vi "Test_Drive_Motor.vi"() -> ()   [LabVIEW 2019]
uses:
  <vilib>/myRIO/Instrument Drivers/Onboard IO/DIO/typedefs/DIO Reference.ctl
  <vilib>/myRIO/Common/Instrument Driver Framework/Utilities/typedefs/myRIO Generic Hardware Reference.ctl
  <vilib>/myRIO/Common/Instrument Driver Framework/Utilities/typedefs/Hardware Version Enum.ctl
  <vilib>/myRIO/Common/Instrument Driver Framework/Utilities/typedefs/myRIO v1.0 Reference.ctl
  <vilib>/myRIO/Common/Instrument Driver Framework/Utilities/typedefs/Generic FPGA Reference.ctl
  <vilib>/myRIO/Common/Instrument Driver Framework/myRIO v1.0/DIO/typedefs/DIO Channels List.ctl
  <vilib>/myRIO/Common/Instrument Driver Framework/myRIO v1.0/DIO/typedefs/DIO Channels Enum.ctl
  <vilib>/userDefined/High Color/nirio_resource_hc.ctl
  L298N_Driver/L298N_Ref_Type.ctl
  L298N_Driver/L298N_Action_Enum.ctl
  <vilib>/myRIO/Common/Instrument Driver Framework/myRIO v1.0/DIO/vis/myRIO v1.1 Open DIO.vi
  <vilib>/myRIO/Common/Instrument Driver Framework/Utilities/vis/Validate Channels.vi
  <vilib>/myRIO/Common/Instrument Driver Framework/myRIO v1.0/DIO/vis/myRIO v1.0 Reserve DIO.vi
  <vilib>/myRIO/Common/Instrument Driver Framework/myRIO v1.0/DIO/vis/myRIO v1.0 Close DIO.vi
  <vilib>/myRIO/Common/Instrument Driver Framework/myRIO v1.0/Resource Manager/vis/myRIO v1.0 Reserve Channel List.vi
  <vilib>/myRIO/Common/Instrument Driver Framework/myRIO v1.0/DIO/vis/myRIO v1.0 Build MUX Configuration DIO.vi
  <vilib>/myRIO/Common/Instrument Driver Framework/myRIO v1.0/DIO/vis/myRIO v1.0 Unreserve DIO.vi
  <vilib>/myRIO/Common/Instrument Driver Framework/myRIO v1.0/Resource Manager/vis/myRIO v1.0 Reserve Channel.vi
  <vilib>/myRIO/Common/Instrument Driver Framework/myRIO v1.0/Resource Manager/vis/myRIO v1.0 Unreserve Channel.vi
  <vilib>/myRIO/Common/Instrument Driver Framework/myRIO v1.0/Resource Manager/vis/myRIO v1.0 Create Configuration List.vi
  <vilib>/myRIO/Common/Instrument Driver Framework/myRIO v1.0/Resource Manager/vis/myRIO v1.0 Unreserve Channel List.vi
  <vilib>/myRIO/Common/Instrument Driver Framework/myRIO v1.0/Resource Manager/vis/myRIO v1.0 Build Mutex Name.vi
  <vilib>/Utility/VariantDataType/GetNumericInfo.vi
  <vilib>/Utility/error.llb/Error Cluster From Error Code.vi
  <vilib>/myRIO/Common/Instrument Driver Framework/myRIO v1.0/myRIO v1.1 Open.vi
  <vilib>/myRIO/Common/Instrument Driver Framework/Utilities/vis/IO Manager.vi
  <vilib>/myRIO/Common/Instrument Driver Framework/Utilities/vis/Configuration Manager.vi
  <vilib>/myRIO/Common/Instrument Driver Framework/myRIO v1.0/Resource Manager/vis/myRIO v1.0 Configure IO.vi
  <vilib>/myRIO/Common/Instrument Driver Framework/myRIO v1.0/myRIO v1.0 Close.vi
  <vilib>/myRIO/Common/Instrument Driver Framework/myRIO v1.0/DIO/vis/myRIO v1.0 Shutdown DIO.vi
  <vilib>/myRIO/Instrument Drivers/Onboard IO/DIO/vis/myRIO DIO Open.xnode
  <vilib>/myRIO/Instrument Drivers/Onboard IO/DIO/DIO.lvlib
panel:
  out "error out":errorcluster caption="sortie d'erreur"
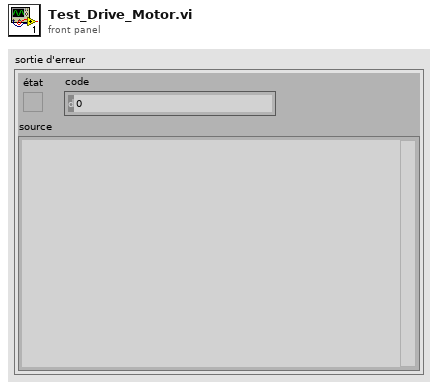
[diagram p1: front panel]
types:
  T1 = typedef "DIO.lvlib/DIO Reference.ctl" = cluster{"myRIO Reference":T2, "DIO Channels List":T6}
  T2 = typedef "myRIO Generic Hardware Reference.ctl" = cluster{"myRIO Model":T3, "myRIO Hardware Reference":T4}
  T3 = typedef "Hardware Version Enum.ctl" = enum16{"Unknown", "myRIO-1900", "myRIO-1950", "roboRIO", "NI ELVIS RIO CM", "ELVIS III"}
  T4 = typedef "myRIO v1.0 Reference.ctl" = cluster{"Generic FPGA Reference":T5, "Allow multiple opens":bool}
  T5 = typedef "Generic FPGA Reference.ctl" = refnum<k20>
  T6 = typedef "DIO Channels List.ctl" = T7[]
  T7 = typedef "DIO Channels Enum.ctl" = enum16{"Not Connected", "C/DIO0", "C/DIO1", "C/DIO2", "C/DIO3", "C/DIO4", "C/DIO5", "C/DIO6", "C/DIO7", "A/DIO0", "A/DIO1", "A/DIO2", "A/DIO3", "A/DIO4", "A/DIO5", "A/DIO6", "A/DIO7", "A/DIO8", "A/DIO9", "A/DIO10", "A/DIO11", "A/DIO12", "A/DIO13", "A/DIO14", "A/DIO15", "A/DIO16", "A/DIO17", "A/DIO18", "A/DIO19", "B/DIO0", "B/DIO1", "B/DIO2", "B/DIO3", "B/DIO4", "B/DIO5", "B/DIO6", "B/DIO7", "B/DIO8", "B/DIO9", "B/DIO10", "B/DIO11", "B/DIO12", "B/DIO13", "B/DIO14", "B/DIO15", "B/DIO16", "B/DIO17", "B/DIO18", "B/DIO19", "LED0", "LED1", "LED2", "LED3", "Button0", "DIO/DIO0", "DIO/DIO1", "DIO/DIO2", "DIO/DIO3", "DIO/DIO4", "DIO/DIO5", "DIO/DIO6", "DIO/DIO7", "DIO/DIO8", "DIO/DIO9", "SPI/CS0", "SPI/CS1", "SPI/CS2", "SPI/CS3", "LED RADIO (Green)", "LED RADIO (Red)", "LED COMM (Green)", "LED COMM (Red)", "LED MODE (Green)", "LED MODE (Red)"}
  T8 = typedef "L298N_Action_Enum.ctl" = enum16{"Monter", "Descendre", "Arreter"}
  T9 = typedef "L298N_Ref_Type.ctl" = cluster{"DIO_Ref_Montee":T1, "DIO_Ref_Descente":T1}
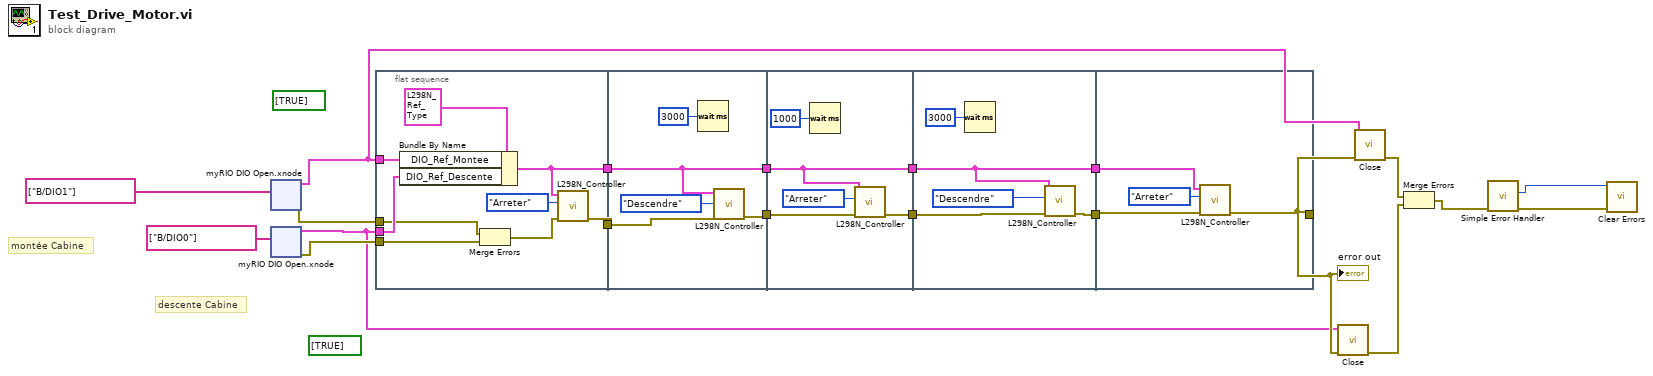
[diagram p0: block diagram]
diagram:
  (unwired) bool[] [TRUE] ("Values")
  (unwired) bool[] [TRUE] ("Values")
  # "montée Cabine"
  # "descente Cabine"
  n1 = xnode "myRIO DIO Open.xnode"("Channel Names"=tag[] ["B/DIO1"]) -> ("error out"=w13:errorcluster, "DIO Ref Out"=w8:T1)  [unwired: 2 in]
  n2 = xnode "myRIO DIO Open.xnode"("Channel Names"=tag[] ["B/DIO0"]) -> ("error out"=w12:errorcluster, "DIO Ref Out"=w7:T1)  [unwired: 2 in]
  n3 = flat-sequence {
    tunnel: w8 -> [w27]
    tunnel: w7 -> [w26]
    tunnel: w13 -> [w25]
    tunnel: w12 -> [w24]
    tunnel: [w22] -> w10
    tunnel: [w21] -> w9
    tunnel: w10 -> [w34]
    tunnel: w9 -> [w30]
    tunnel: [w32] -> w5
    tunnel: [w30] -> w4
    tunnel: w5 -> [w39]
    tunnel: w4 -> [w37]
    tunnel: [w37] -> w3
    tunnel: [w38] -> w2
    tunnel: w3 -> [w43]
    tunnel: [w43] -> w6
    tunnel: w2 -> [w44]
    tunnel: [w40] -> w1
    tunnel: [w47] -> w11
    tunnel: w6 -> [w46]
    tunnel: w1 -> [w48]
    frame #0 {
      n4 = Bundle By Name(cluster=T9 {"DIO_Ref_Montee"={"myRIO Reference"={"myRIO Model"=enum."myRIO-1900", "myRIO Hardware Reference"={"Generic FPGA Reference"=refnum, "Allow multiple opens"=FALSE}}, "DIO Channels List"=[]}, "DIO_Ref_Descente"={"myRIO Reference"={"myRIO Model"=enum."myRIO-1900", "myRIO Hardware Reference"={"Generic FPGA Reference"=refnum, "Allow multiple opens"=FALSE}}, "DIO Channels List"=[]}} ("Cluster"), "DIO_Ref_Montee"=w27, "DIO_Ref_Descente"=w26) -> (w21:T9)
      n5 = Merge Errors(w25, w24) -> (w29:errorcluster)
      n6 = call "L298N_Controller.vi"("Error In"=w29, "Action_Moteur"=L298N_Action_Enum."Arreter", "Cluster"=w21) -> ("Error Out"=w22:errorcluster)  [unwired: 8 in]
    }
    frame #1 {
      n7 = Wait (ms)(milliseconds to wait=u32 3000 ("attente (ms)")) -> ()  [unwired: 1 out]
      n8 = call "L298N_Controller.vi"("Error In"=w34, "Action_Moteur"=L298N_Action_Enum."Descendre", "Cluster"=w30) -> ("Error Out"=w32:errorcluster)  [unwired: 8 in]
    }
    frame #2 {
      n9 = Wait (ms)(milliseconds to wait=u32 1000 ("attente (ms)")) -> ()  [unwired: 1 out]
      n10 = call "L298N_Controller.vi"("Error In"=w39, "Action_Moteur"=L298N_Action_Enum."Arreter", "Cluster"=w37) -> ("Error Out"=w38:errorcluster)  [unwired: 8 in]
    }
    frame #3 {
      n11 = Wait (ms)(milliseconds to wait=u32 3000 ("attente (ms)")) -> ()  [unwired: 1 out]
      n12 = call "L298N_Controller.vi"("Error In"=w44, "Action_Moteur"=L298N_Action_Enum."Descendre", "Cluster"=w43) -> ("Error Out"=w40:errorcluster)  [unwired: 8 in]
    }
    frame #4 {
      n13 = call "L298N_Controller.vi"("Error In"=w48, "Action_Moteur"=L298N_Action_Enum."Arreter", "Cluster"=w46) -> ("Error Out"=w47:errorcluster)  [unwired: 8 in]
    }
  }
  n14 = call <vilib>:"Close.vi"("error in (no error)"=w11, "DIO Ref In"=w7) -> ("error out"=w15:errorcluster)  [unwired: 9 in]
  n15 = call <vilib>:"Close.vi"("error in (no error)"=w11, "DIO Ref In"=w8) -> ("error out"=w16:errorcluster)  [unwired: 9 in]
  n16 = Merge Errors(w16, w15) -> (w14:errorcluster)
  n17 = call <vilib>:"Simple Error Handler.vi"("error in (no error)"=w14) -> ("code out"=w17:i32, "error out"=w18:errorcluster)  [unwired: 4 in, 3 out]
  n18 = call <vilib>:"Clear Errors.vi"("error in (no error)"=w18, "specific error code to clear (0: all)"=w17) -> ()  [unwired: 4 in, 2 out]
  "error out" <- w11
